vi "verify errors.vi"(8 "error in (no error)":errorcluster, 11 "Channel in":refnum<class "Channel.lvclass">) -> (0 "error out":errorcluster, 2 "error":bool, 3 "Channel out":refnum<class "Channel.lvclass">)   [LabVIEW 2018, in "Channel.lvclass"]
uses:
  Channel.lvclass
  Channel.lvclass/Channel.ctl
  Sim_CCD/Sim_CCD.lvclass/Sim_CCD.ctl
  Sim_CCD/Sim_CCD.lvclass
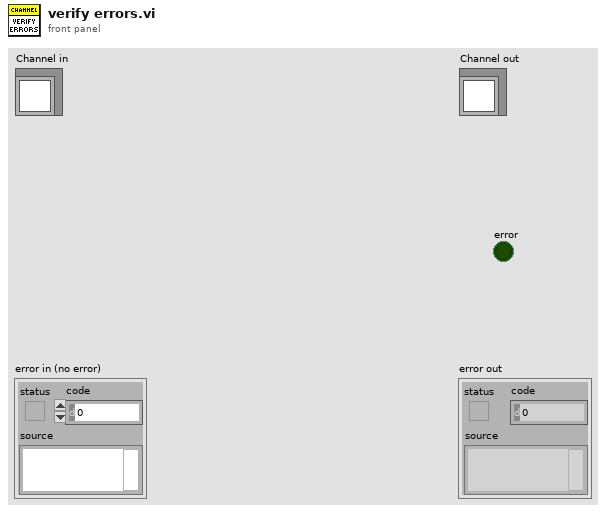
[diagram p1: front panel]
types:
  T1 = cluster{"EXPTIME":errorcluster, "#FRAMES":errorcluster}
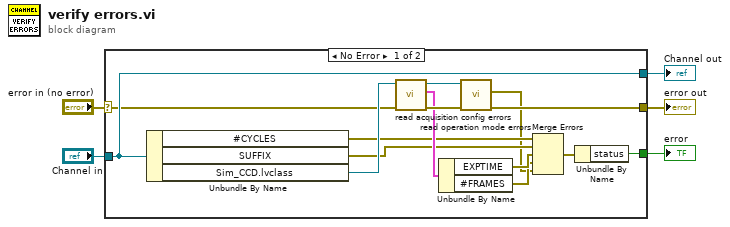
[diagram p0: block diagram]
diagram:
  n1 = case shown="No Error" "error in (no error)" {
    selector: "error in (no error)" -> [w17 w21]
    tunnel: [w14 w21] -> w4
    tunnel: [w19 w20] -> w2
    tunnel: "Channel in" -> [w19 w20]
    tunnel: [w6 _] -> w1
    frame No Error {
      n2 = Unbundle By Name(w19) -> ("#CYCLES"=w12:errorcluster, "SUFFIX"=w11:errorcluster, "Sim_CCD.lvclass"=w18:refnum<class "Sim_CCD.lvclass">)
      n3 = call "read acquisition config errors.vi"("error in (no error)"=w17, "Simulated Camera in"=w18) -> ("error out"=w16:errorcluster, "acq config errors"=w13:T1, "Simulated Camera out"=w15:refnum<class "Sim_CCD.lvclass">)  [unwired: 7 in]
      n4 = Unbundle By Name(w13) -> ("EXPTIME"=w10:errorcluster, "#FRAMES"=w9:errorcluster)
      n5 = call "read operation mode errors.vi"("error in (no error)"=w16, "Simulated_CCD_Camera in"=w15) -> ("error out"=w14:errorcluster, "WRITE SETUP errors"=w8:errorcluster[])  [unwired: 7 in, 1 out]
      n6 = Merge Errors(w12, w11, w10, w9, w8) -> (w7:errorcluster)
      n7 = Unbundle By Name(w7) -> ("status"=w6:bool)
    }
    frame Error {
    }
  }
  "error out" <- w4
  "Channel out" <- w2
  "error" <- w1
